vi "open usb.vi"(7 "altiface":i32, 9 "iface":i32, 10 "conf":i32, 11 "idx":i32) -> (3 "function return":i32)   [LabVIEW 2013, in "libusvlv.lvlib"]
doc: "extern \"C\" int _declspec_dll_use open_usb(int idx, int conf, int iface, int altiface);"
uses:
  libusvlv.lvlib
  UsbCom.dll
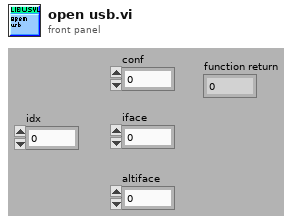
[diagram p1: front panel]
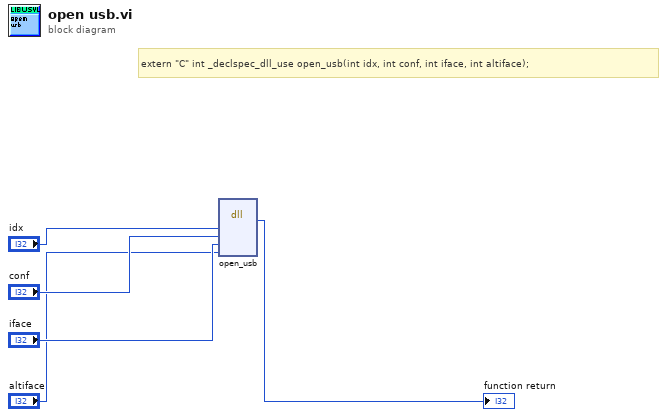
[diagram p0: block diagram]
diagram:
  # "extern \"C\" int _declspec_dll_use open_usb(int idx, int conf, int iface, int altiface);"
  n1 = dll-call lib="E:/libusvlv/UsbCom.dll" fn="open_usb"("idx"="idx", "conf"="conf", "iface"="iface", "altiface"="altiface") -> ("返回类型"=→"function return":i32)  [unwired: 7 in, 2 out]
